vi "FTW-Actor-HandleError.vi"(0 "FTW Actor Instance":refnum<class "FTW-Actor-Instance.lvclass">, 5 "Explanation":string, 11 "error in":errorcluster) -> (4 "FTW Actor Instance out":refnum<class "FTW-Actor-Instance.lvclass">, 6 "Exception occured?":T1, 15 "error out":errorcluster)   [LabVIEW 2014, in "FTW-Actor-Instance.lvclass"]
uses:
  FTW-Actor-Instance.lvclass
  error/FTW-ERR-ExceptionType.ctl
panel:
  # "Inputs"
  # "Outputs"
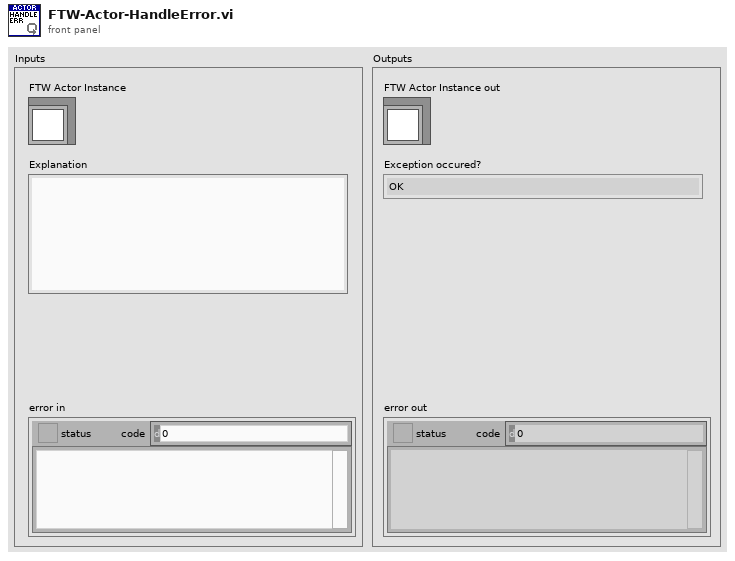
[diagram p1: front panel]
types:
  T1 = typedef "FTW-ERR-ExceptionType.ctl" = enum16{"OK", "Info", "Warning", "Error"}
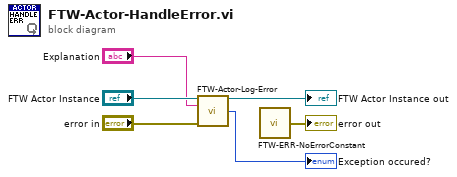
[diagram p0: block diagram]
diagram:
  n1 = call-dynamic "FTW-Actor-Log-Error.vi"("FTW Actor Instance"="FTW Actor Instance", "Explanation"="Explanation", "Error to Log"="error in") -> ("FTW Actor Instance out"=→"FTW Actor Instance out":refnum<class "FTW-Actor-Instance.lvclass">, "Exception"=→"Exception occured?":T1)  [unwired: 10 in, 1 out]
  n2 = call "FTW-ERR-NoErrorConstant.vi"() -> ("no error"=→"error out":errorcluster)
